vi "Get Cell Data Type.vi"(0 "object in":refnum<class "Spreadsheet.lvclass">, 1 "Cell":T1, 5 "error in (no error)":errorcluster) -> (14 "object out":refnum<class "Spreadsheet.lvclass">, 15 "ReturnedData":string[][](array[string]), 19 "error out":errorcluster)   [LabVIEW 2013, in "Spreadsheet.lvclass"]
uses:
  Spreadsheet.lvclass
  Cell.ctl
  Spreadsheet.lvclass/Spreadsheet.ctl
panel:
  # "Input"
  # "Output"
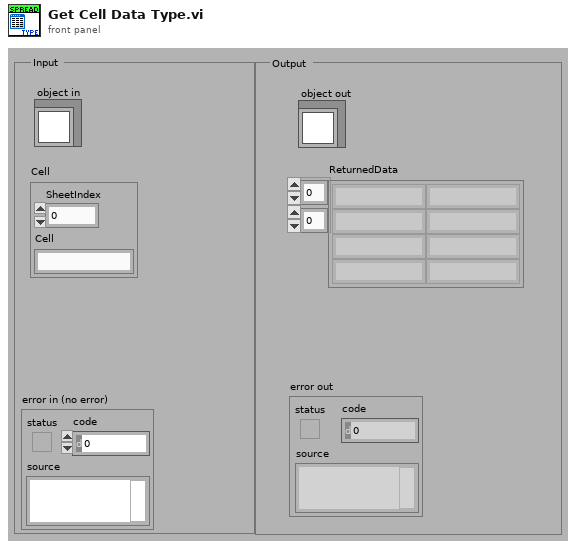
[diagram p1: front panel]
types:
  T1 = typedef "Cell.ctl" = cluster{"SheetIndex":u8, "Cell":string}
  T2 = cluster{"Table Data":string[][], "Cell Info":string[][], "SheetName":string}[]
  T3 = cluster{"Table Data":string[][], "Cell Info":string[][], "SheetName":string}
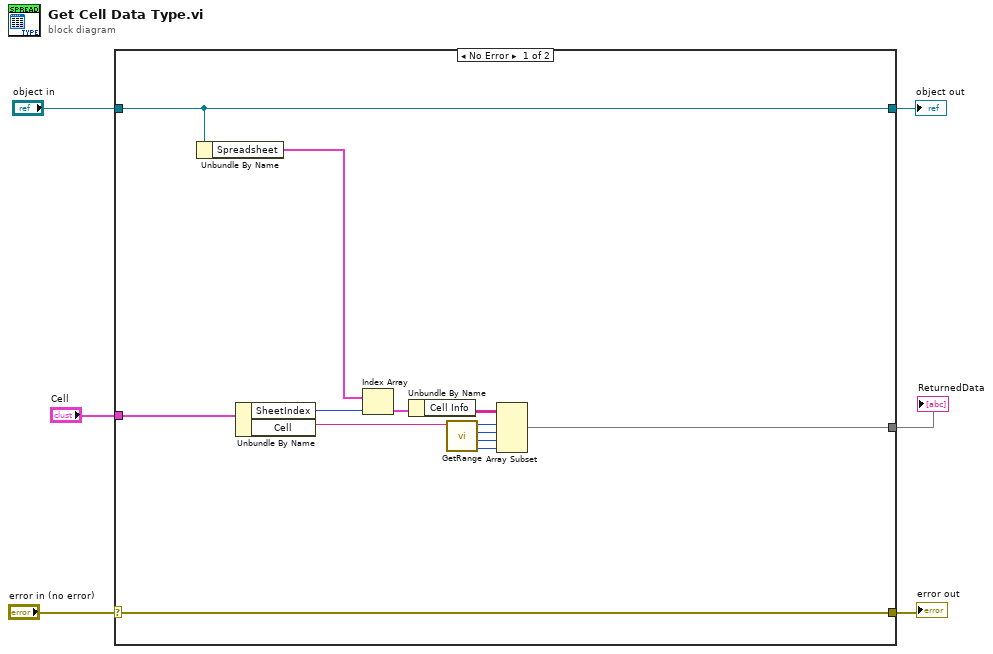
[diagram p0: block diagram]
diagram:
  n1 = case shown="No Error" "error in (no error)" {
    selector: "error in (no error)" -> [w19 w21]
    tunnel: [w19 w21] -> w5
    tunnel: [w18 w20] -> w3
    tunnel: "object in" -> [w18 w20]
    tunnel: "Cell" -> [w8 _]
    tunnel: [w7 _] -> w1
    frame No Error {
      n2 = Unbundle By Name(w18) -> ("Spreadsheet"=w9:T2)
      n3 = Unbundle By Name(w8) -> ("SheetIndex"=w15:u8, "Cell"=w14:string)
      n4 = Index Array(array=w9, index=w15) -> (element=w17:T3)
      n5 = Unbundle By Name(w17) -> ("Cell Info"=w16:string[][])
      n6 = call "GetRange.vi"("String"=w14) -> ("#Col Elements"=w10:i32, "Start Column"=w12:i32, "#RowElements"=w11:i32, "Start Row"=w13:i32)  [unwired: 7 in]
      n7 = Array Subset(array=w16, index (row)=w13, length (row)=w11, index (col)=w12, length (col)=w10) -> (w7:string[][])
    }
    frame Error {
    }
  }
  "error out" <- w5
  "object out" <- w3
  "ReturnedData" <- w1
